vi "Launch Action - XNET CAN Readers with ID.vi"(7 "PackageID":i32, 8 "error in (no error)":errorcluster, 11 "CAN Configuration":T1={"CAN Interface"="CAN1", "XNET Cluster"="ManyXnetChannels", "#Signals"=0, "Sample Rate (Hz)"=100.0} {"Sample Rate (Hz)" format="%#_13g"}) -> (0 "error out":errorcluster)   [LabVIEW 2021, in "XNET-CAN-Signal-Logger.lvlib"]
uses:
  XNET-CAN-Signal-Logger.lvlib
  Typedef/Def-CAN Port Configuration.ctl
  Action - XNET CAN Reader with ID.vi
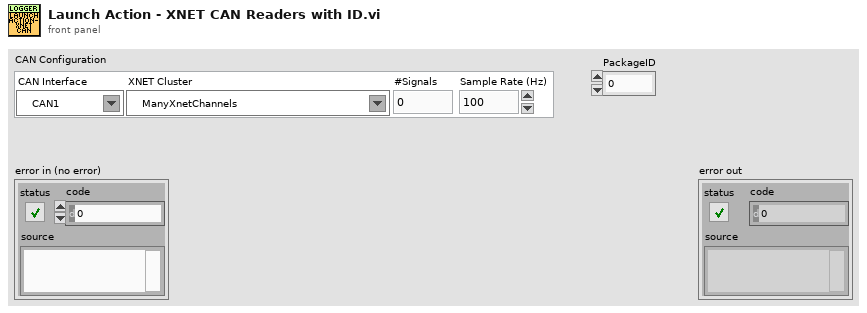
[diagram p1: front panel]
types:
  T1 = typedef "XNET-CAN-Signal-Logger.lvlib/Def-CAN Port Configuration.ctl" = cluster{"CAN Interface":refnum<k21>, "XNET Cluster":refnum<k21>, "#Signals":i32, "Sample Rate (Hz)":dbl}
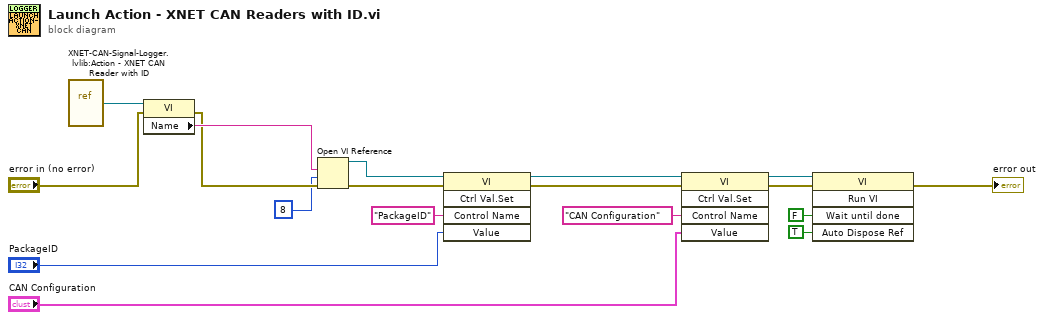
[diagram p0: block diagram]
diagram:
  n1 = vi-ref "XNET-CAN-Signal-Logger.lvlib:Action - XNET CAN Reader with ID.vi"() -> (w18:refnum<vi>)
  n2 = property class="VI"(reference=w18, error in="error in (no error)") -> (error out=w15:errorcluster, "Name"=w17:string)  [unwired: 1 out]
  n3 = Open VI Reference(vi path=w17, options=8, error in (no error)=w15) -> (vi reference=w4:refnum<vi>, error out=w5:errorcluster)  [unwired: 3 in]
  n4 = invoke class="VI" method="Ctrl Val.Set"(reference=w4, error in=w5, "Control Name"="PackageID", "Value"="PackageID") -> (reference out=w3:refnum<vi>, error out=w2:errorcluster)  [unwired: 1 in, 3 out]
  n5 = invoke class="VI" method="Ctrl Val.Set"(reference=w3, error in=w2, "Control Name"="CAN Configuration", "Value"="CAN Configuration") -> (reference out=w10:refnum<vi>, error out=w9:errorcluster)  [unwired: 1 in, 3 out]
  n6 = invoke class="VI" method="Run VI"(reference=w10, error in=w9, "Wait until done"=FALSE ("Wait Until Done"), "Auto Dispose Ref"=TRUE ("Auto Dispose Reference")) -> (error out=→"error out":errorcluster)  [unwired: 1 in, 4 out]
